vi "Write Card Arr Ref.vi"(8 "error in (no error)":errorcluster, 10 "Card Arr Ref":refnum<vi>, 11 "Generic Instrument in":refnum<class "Generic Instrument.lvclass">) -> (0 "error out":errorcluster, 3 "Generic Instrument out":refnum<class "Generic Instrument.lvclass">)   [LabVIEW 2016, in "Generic Instrument.lvlib" / "Generic Instrument.lvclass"]
uses:
  Generic Instrument.lvclass
  Generic Instrument.lvclass/Generic Instrument.ctl
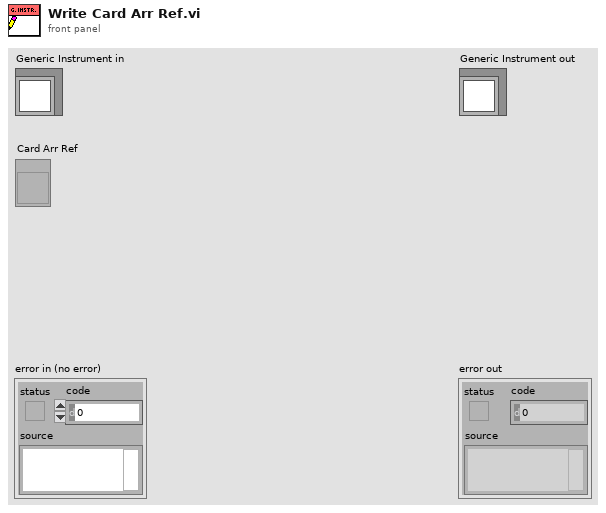
[diagram p1: front panel]
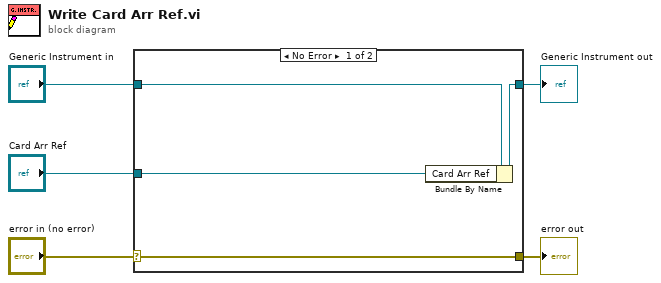
[diagram p0: block diagram]
diagram:
  n1 = case shown="No Error" "error in (no error)" {
    selector: "error in (no error)" -> [w9 w10]
    tunnel: [w9 w10] -> w4
    tunnel: [w7 w11] -> w2
    tunnel: "Generic Instrument in" -> [w8 w11]
    tunnel: "Card Arr Ref" -> [w6 _]
    frame No Error {
      n2 = Bundle By Name(cluster=w8, "Card Arr Ref"=w6) -> (w7:refnum<class "Generic Instrument.lvclass">)
    }
    frame Error {
    }
  }
  "error out" <- w4
  "Generic Instrument out" <- w2
